vi "Pkt - Export Channel Configuration.vi"(8 "error in (no error)":errorcluster, 11 "Channel Config Data":T1) -> (0 "error out":errorcluster)   [LabVIEW 2019, in "UDP-Custom-Device System Explorer.lvlib"]
uses:
  UDP-Custom-Device System Explorer.lvlib
  Types/Channel Configuration/Channel Config File Data.ctl
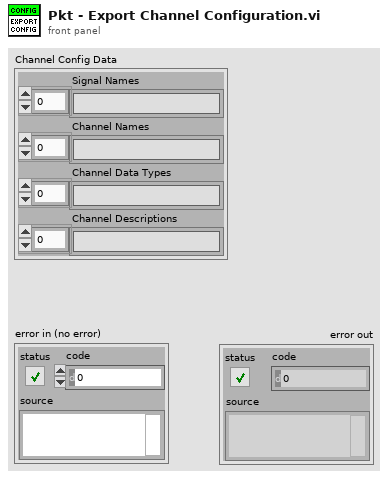
[diagram p1: front panel]
types:
  T1 = typedef "UDP-Custom-Device System Explorer.lvlib/Channel Config File Data.ctl" = cluster{"Signal Names":string[], "Channel Names":string[], "Channel Data Types":string[], "Channel Descriptions":string[]}
  T2 = enum16{"open", "replace", "create", "open or create", "replace or create", "replace or create with confirmation"}
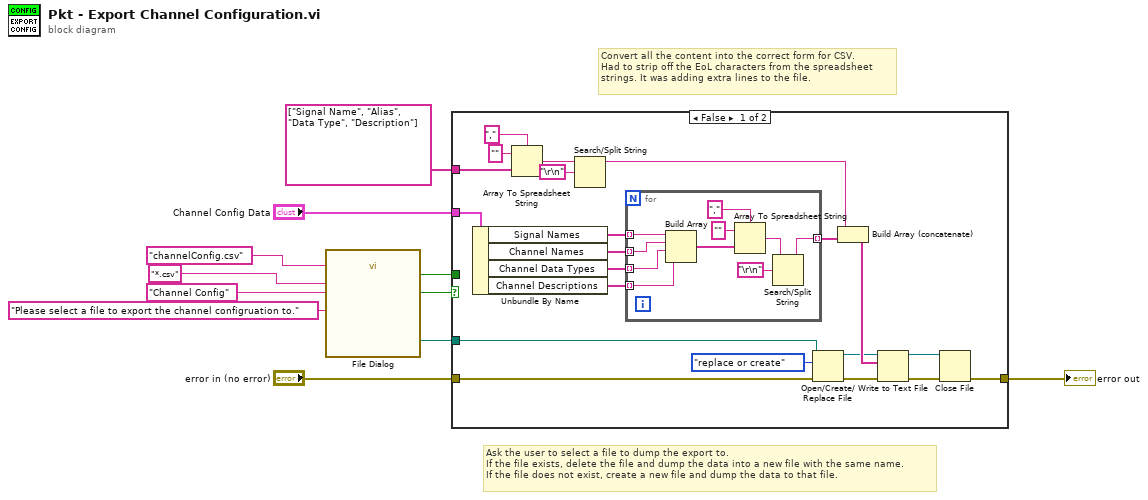
[diagram p0: block diagram]
diagram:
  # "Convert all the content into the correct form for CSV.\nHad to strip off the EoL characters from the spreadsheet\nstrings. It was adding extra lines to the file."
  # "Ask the user to select a file to dump the export to.\nIf the file exists, delete the file and dump the data into a new file with the same name.\nIf the file does not exist, create a new file and dump the data to that file."
  n1 = call "File Dialog"("prompt"="Please select a file to export the channel configruation to.", "default name"="channelConfig.csv", "pattern (all files)"="*.csv", "pattern label"="Channel Config") -> ("selected path"=w6:path, "exists"=w2:bool, "cancelled"=w7:bool)  [unwired: 8 in, 1 out]
  n2 = case shown="False" w7 {
    tunnel: w6 -> [w32 _]
    tunnel: "Channel Config Data" -> [w29 _]
    tunnel: [w16 w43] -> w4
    tunnel: "error in (no error)" -> [w31 w43]
    tunnel: w2 -> [_ _]
    tunnel: string[] ["Signal Name", "Alias", "Data Type", "Description"] ("element") -> [w26 _]
    frame False {
      n3 = Unbundle By Name(w29) -> ("Signal Names"=w25:string[], "Channel Names"=w24:string[], "Channel Data Types"=w23:string[], "Channel Descriptions"=w22:string[])
      n4 = Array To Spreadsheet String(delimiter (Tab)=",", array=w26, 3:"" ("format string")) -> (spreadsheet string=w13:string)
      n5 = Search/Split String(string=w13, search string/char (-)="\r\n") -> (substring before match=w12:string)  [unwired: 1 in, 2 out]
      n6 = for {
        tunnel: w25 -> [w40] mode=indexing
        tunnel: w24 -> [w39] mode=indexing
        tunnel: w23 -> [w38] mode=indexing
        tunnel: w22 -> [w37] mode=indexing
        tunnel: [w33] -> w21 mode=indexing
        n7 = Build Array(w40, w39, w38, w37) -> (w36:string[])
        n8 = Array To Spreadsheet String(delimiter (Tab)=",", array=w36, 3:"" ("format string")) -> (spreadsheet string=w34:string)
        n9 = Search/Split String(string=w34, search string/char (-)="\r\n") -> (substring before match=w33:string)  [unwired: 1 in, 2 out]
      }
      n10 = Open/Create/Replace File(file path (use dialog)=w32, error in=w31, operation (0:open)=T2."replace or create") -> (refnum out=w19:refnum<file>, error out=w18:errorcluster)  [unwired: 3 in, 1 out]
      n11 = Build Array (concatenate)(w12, w21) -> (w20:string[])
      n12 = Write to Text File(file (use dialog)=w19, text=w20, error in=w18) -> (refnum out=w15:refnum<file>, error out=w17:errorcluster)  [unwired: 1 in, 1 out]
      n13 = Close File(refnum=w15, error in=w17) -> (error out=w16:errorcluster)  [unwired: 1 out]
    }
    frame True {
      # "Cancelled. Do nothing."
    }
  }
  "error out" <- w4
